vi "Initialize.vi"(7 "Component ID (1-8)":u8=1, 8 "error in (no error)":errorcluster, 9 "SubComponents":refnum<class "1553 SubComponent.lvclass">[](array[class]), 10 "FPGA Interface":refnum<class "FPGA Interface.lvclass">) -> (0 "error out":errorcluster, 3 "1553 Component out":refnum<class "1553 Component.lvclass">)   [LabVIEW 2020, in "BCI-1553 API.lvlib" / "1553 Component.lvclass"]
doc: "Initializes a component. The Component ID is the FPGA Reference location of the BCI-1553 module in a chassis. The FPGA interface is required for communication to the physical hardware. The subcomponents dictate the specific behavior of this component. A Component can simultaneously support:\n\n1 Bus Controller\n1 Bus Monitor\n2 Remote Terminals\n\nAny smaller mix of these SubComponents is also valid. Please note that any Bus Monitor SubComponent will automatically rearrange itself to be the last SubComponent in the list."
uses:
  1553 Component.lvclass
  1553 SubComponent/1553 SubComponent.lvclass
  Dependencies/FPGA Interface/FPGA Interface.lvclass
  1553 Component.lvclass/1553 Component.ctl
  Dependencies/Virtual Memory Unit/Virtual Memory Unit.lvclass
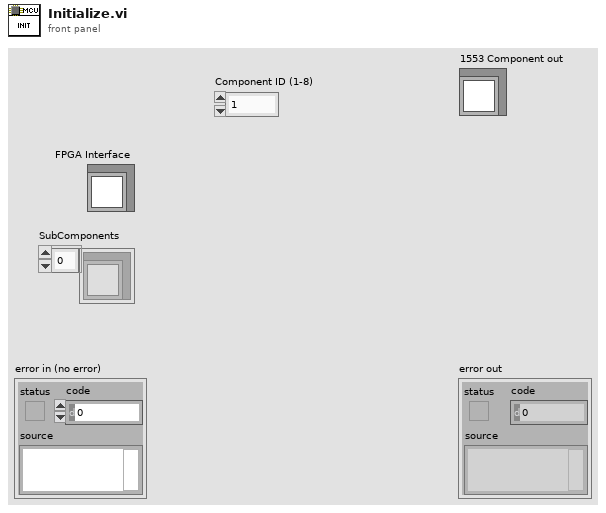
[diagram p1: front panel]
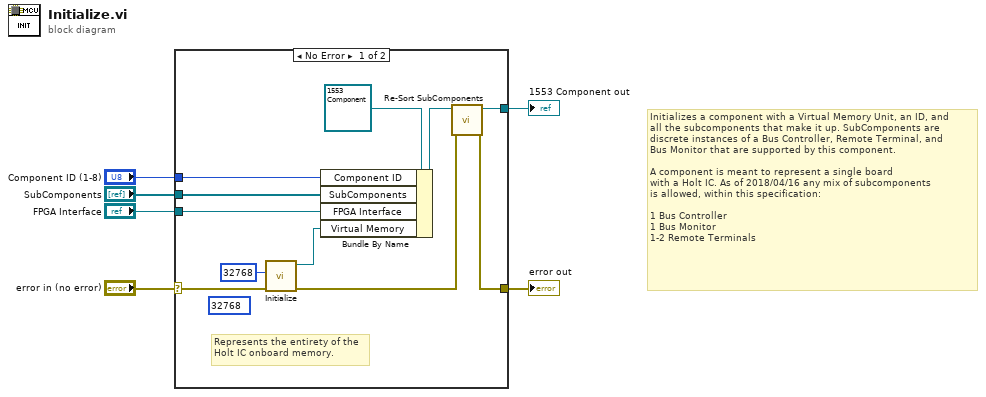
[diagram p0: block diagram]
diagram:
  # "Initializes a component with a Virtual Memory Unit, an ID, and\nall the subcomponents that make it up. SubComponents are\ndiscrete instances of a Bus Controller, Remote Terminal, and\nBus Monitor that are supported by this component.\n\nA component is meant to represent a single board\nwith a Holt IC. As of 2018/04/16 any mix of subcomponents\nis allowed, within this specification:\n\n1 Bus Controller\n1 Bus Monitor\n1-2 Remote Terminals"
  n1 = case shown="No Error" "error in (no error)" {
    selector: "error in (no error)" -> [w13 w18]
    tunnel: [w7 w18] -> w5
    tunnel: [w9 _] -> w4
    tunnel: "Component ID (1-8)" -> [w16 _]
    tunnel: "SubComponents" -> [w15 _]
    tunnel: "FPGA Interface" -> [w11 _]
    frame No Error {
      (unwired) 32768 ("Memory Size")
      # "Represents the entirety of the\nHolt IC onboard memory."
      n2 = call "Initialize.vi"("error in (no error)"=w13, "Memory Size"=32768) -> ("error out"=w8:errorcluster, "Virtual Memory Unit out"=w14:refnum<class "Virtual Memory Unit.lvclass">)  [unwired: 8 in]
      n3 = Bundle By Name(cluster=refnum<class "1553 Component.lvclass"> refnum ("1553 Component in"), "Component ID"=w16, "SubComponents"=w15, "FPGA Interface"=w11, "Virtual Memory"=w14) -> (w10:refnum<class "1553 Component.lvclass">)
      n4 = call "Re-Sort SubComponents.vi"("error in (no error)"=w8, "1553 Component in"=w10) -> ("error out"=w7:errorcluster, "1553 Component out"=w9:refnum<class "1553 Component.lvclass">)  [unwired: 8 in]
    }
    frame Error {
    }
  }
  "error out" <- w5
  "1553 Component out" <- w4
